vi "Language.vi"(6 "language cmd":T2, 8 "error in (no error)":errorcluster, 9 "Language":T3) -> (0 "error out":errorcluster, 3 "Language Data out":T1)   [LabVIEW 2015, in "AguaClara Library.lvlib"]
uses:
  AguaClara Library.lvlib
  Language.ctl
  language cmd.ctl
  Variable cluster.ctl
panel:
  in  "Language Data storage":T1=[{"Label.Text"="Quit", "Control Type"=0, "Numeric"=0.0, "Array"=[], "status"=FALSE, "Str Array"=[], "String"="", "unit"=""}, {"Label.Text"="Tab Control", "Control Type"=0, "Numeric"=0.0, "Array"=[], "status"=FALSE, "Str Array"=[], "String"="", "unit"=""}, {"Label.Text"="Help Button", "Control Type"=0, "Numeric"=0.0, "Array"=[], "status"=FALSE, "Str Array"=[], "String"="", "unit"=""}, {"Label.Text"="Logon", "Control Type"=0, "Numeric"=0.0, "Array"=[], "status"=FALSE, "Str Array"=[], "String"="", "unit"=""}, {"Label.Text"="Project List", "Control Type"=0, "Numeric"=0.0, "Array"=[], "status"=FALSE, "Str Array"=[], "String"="", "unit"=""}, {"Label.Text"="Project commands", "Control Type"=0, "Numeric"=0.0, "Array"=[], "status"=FALSE, "Str Array"=[], "String"="", "unit"=""}, {"Label.Text"="Log off", "Control Type"=0, "Numeric"=0.0, "Array"=[], "status"=FALSE, "Str Array"=[], "String"="", "unit"=""}, {"Label.Text"="Design Plant", "Control Type"=0, "Numeric"=0.0, "Array"=[], "status"=FALSE, "Str Array"=[], "String"="", "unit"=""}, {"Label.Text"="Project Info label", "Control Type"=0, "Numeric"=0.0, "Array"=[], "status"=FALSE, "Str Array"=[], "String"="", "unit"=""}, {"Label.Text"="Design Inputs Label", "Control Type"=0, "Numeric"=0.0, "Array"=[], "status"=FALSE, "Str Array"=[], "String"="", "unit"=""}, {"Label.Text"="MSG Design sent precity", "Control Type"=0, "Numeric"=0.0, "Array"=[], "status"=FALSE, "Str Array"=[], "String"="", "unit"=""}, {"Label.Text"="MSG Design sent postcity", "Control Type"=0, "Numeric"=0.0, "Array"=[], "status"=FALSE, "Str Array"=[], "String"="", "unit"=""}, {"Label.Text"="MSG Server unavailable", "Control Type"=0, "Numeric"=0.0, "Array"=[], "status"=FALSE, "Str Array"=[], "String"="", "unit"=""}, {"Label.Text"="Quit now", "Control Type"=0, "Numeric"=0.0, "Array"=[], "status"=FALSE, "Str Array"=[], "String"="", "unit"=""}, {"Label.Text"="Project Info", "Control Type"=0, "Numeric"=0.0, "Array"=[], "status"=FALSE, "Str Array"=[], "String"="", "unit"=""}, {"Label.Text"="Project Name", "Control Type"=0, "Numeric"=0.0, "Array"=[], "status"=FALSE, "Str Array"=[], "String"="", "unit"=""}, {"Label.Text"="City", "Control Type"=0, "Numeric"=0.0, "Array"=[], "status"=FALSE, "Str Array"=[], "String"="", "unit"=""}, {"Label.Text"="State", "Control Type"=0, "Numeric"=0.0, "Array"=[], "status"=FALSE, "Str Array"=[], "String"="", "unit"=""}, {"Label.Text"="Country", "Control Type"=0, "Numeric"=0.0, "Array"=[], "status"=FALSE, "Str Array"=[], "String"="", "unit"=""}, {"Label.Text"="Notes", "Control Type"=0, "Numeric"=0.0, "Array"=[], "status"=FALSE, "Str Array"=[], "String"="", "unit"=""}, {"Label.Text"="User Information", "Control Type"=0, "Numeric"=0.0, "Array"=[], "status"=FALSE, "Str Array"=[], "String"="", "unit"=""}, {"Label.Text"="First Name", "Control Type"=0, "Numeric"=0.0, "Array"=[], "status"=FALSE, "Str Array"=[], "String"="", "unit"=""}, {"Label.Text"="Last Name", "Control Type"=0, "Numeric"=0.0, "Array"=[], "status"=FALSE, "Str Array"=[], "String"="", "unit"=""}, {"Label.Text"="Email Address", "Control Type"=0, "Numeric"=0.0, "Array"=[], "status"=FALSE, "Str Array"=[], "String"="", "unit"=""}, {"Label.Text"="Organization", "Control Type"=0, "Numeric"=0.0, "Array"=[], "status"=FALSE, "Str Array"=[], "String"="", "unit"=""}, {"Label.Text"="Language", "Control Type"=0, "Numeric"=0.0, "Array"=[], "status"=FALSE, "Str Array"=[], "String"="", "unit"=""}, {"Label.Text"="AutoCAD File Type", "Control Type"=0, "Numeric"=0.0, "Array"=[], "status"=FALSE, "Str Array"=[], "String"="", "unit"=""}, {"Label.Text"="Project date", "Control Type"=0, "Numeric"=0.0, "Array"=[], "status"=FALSE, "Str Array"=[], "String"="", "unit"=""}, {"Label.Text"="Design Inputs", "Control Type"=0, "Numeric"=0.0, "Array"=[], "status"=FALSE, "Str Array"=[], "String"="", "unit"=""}, {"Label.Text"="Q.Plant", "Control Type"=0, "Numeric"=0.0, "Array"=[], "status"=FALSE, "Str Array"=[], "String"="", "unit"=""}, {"Label.Text"="C.CoagDoseMax", "Control Type"=0, "Numeric"=0.0, "Array"=[], "status"=FALSE, "Str Array"=[], "String"="", "unit"=""}, {"Label.Text"="C.CoagStock", "Control Type"=0, "Numeric"=0.0, "Array"=[], "status"=FALSE, "Str Array"=[], "String"="", "unit"=""}, {"Label.Text"="Ti.CoagStock", "Control Type"=0, "Numeric"=0.0, "Array"=[], "status"=FALSE, "Str Array"=[], "String"="", "unit"=""}, {"Label.Text"="EN.DrillSeries", "Control Type"=0, "Numeric"=0.0, "Array"=[], "status"=FALSE, "Str Array"=[], "String"="", "unit"=""}, {"Label.Text"="EN.TubeSeries", "Control Type"=0, "Numeric"=0.0, "Array"=[], "status"=FALSE, "Str Array"=[], "String"="", "unit"=""}, {"Label.Text"="EN.PipeSeries", "Control Type"=0, "Numeric"=0.0, "Array"=[], "status"=FALSE, "Str Array"=[], "String"="", "unit"=""}, {"Label.Text"="N.SedTanks", "Control Type"=0, "Numeric"=0.0, "Array"=[], "status"=FALSE, "Str Array"=[], "String"="", "unit"=""}, {"Label.Text"="N.SedBaysEst", "Control Type"=0, "Numeric"=0.0, "Array"=[], "status"=FALSE, "Str Array"=[], "String"="", "unit"=""}, {"Label.Text"="W.SedPlate", "Control Type"=0, "Numeric"=0.0, "Array"=[], "status"=FALSE, "Str Array"=[], "String"="", "unit"=""}, {"Label.Text"="L.SedPlateSheet", "Control Type"=0, "Numeric"=0.0, "Array"=[], "status"=FALSE, "Str Array"=[], "String"="", "unit"=""}, {"Label.Text"="T.SedPlate", "Control Type"=0, "Numeric"=0.0, "Array"=[], "status"=FALSE, "Str Array"=[], "String"="", "unit"=""}, {"Label.Text"="T.PlantWall", "Control Type"=0, "Numeric"=0.0, "Array"=[], "status"=FALSE, "Str Array"=[], "String"="", "unit"=""}, {"Label.Text"="H.FlocOption", "Control Type"=0, "Numeric"=0.0, "Array"=[], "status"=FALSE, "Str Array"=[], "String"="", "unit"=""}, {"Label.Text"="T.FlocBaffleRigidH", "Control Type"=0, "Numeric"=0.0, "Array"=[], "status"=FALSE, "Str Array"=[], "String"="", "unit"=""}, {"Label.Text"="T.ConcreteMin", "Control Type"=0, "Numeric"=0.0, "Array"=[], "status"=FALSE, "Str Array"=[], "String"="", "unit"=""}, {"Label.Text"="T.SedWeir", "Control Type"=0, "Numeric"=0.0, "Array"=[], "status"=FALSE, "Str Array"=[], "String"="", "unit"=""}, {"Label.Text"="T.FlocBaffleRigidV", "Control Type"=0, "Numeric"=0.0, "Array"=[], "status"=FALSE, "Str Array"=[], "String"="", "unit"=""}, {"Label.Text"="error out", "Control Type"=0, "Numeric"=0.0, "Array"=[], "status"=FALSE, "Str Array"=[], "String"="", "unit"=""}, {"Label.Text"="status", "Control Type"=0, "Numeric"=0.0, "Array"=[], "status"=FALSE, "Str Array"=[], "String"="", "unit"=""}, {"Label.Text"="code", "Control Type"=0, "Numeric"=0.0, "Array"=[], "status"=FALSE, "Str Array"=[], "String"="", "unit"=""}, {"Label.Text"="source", "Control Type"=0, "Numeric"=0.0, "Array"=[], "status"=FALSE, "Str Array"=[], "String"="", "unit"=""}, {"Label.Text"="File List", "Control Type"=0, "Numeric"=0.0, "Array"=[], "status"=FALSE, "Str Array"=[], "String"="", "unit"=""}, {"Label.Text"="Translate", "Control Type"=0, "Numeric"=0.0, "Array"=[], "status"=FALSE, "Str Array"=[], "String"="", "unit"=""}, {"Label.Text"="CheckOut ADT", "Control Type"=0, "Numeric"=0.0, "Array"=[], "status"=FALSE, "Str Array"=[], "String"="", "unit"=""}, {"Label.Text"="ADT version", "Control Type"=0, "Numeric"=0.0, "Array"=[], "status"=FALSE, "Str Array"=[], "String"="", "unit"=""}, {"Label.Text"="Choose Server", "Control Type"=0, "Numeric"=0.0, "Array"=[], "status"=FALSE, "Str Array"=[], "String"="", "unit"=""}, {"Label.Text"="design server", "Control Type"=0, "Numeric"=0.0, "Array"=[], "status"=FALSE, "Str Array"=[], "String"="", "unit"=""}, {"Label.Text"="Restart ADT", "Control Type"=0, "Numeric"=0.0, "Array"=[], "status"=FALSE, "Str Array"=[], "String"="", "unit"=""}, {"Label.Text"="Create New Project", "Control Type"=0, "Numeric"=0.0, "Array"=[], "status"=FALSE, "Str Array"=[], "String"="", "unit"=""}, {"Label.Text"="Edit Project", "Control Type"=0, "Numeric"=0.0, "Array"=[], "status"=FALSE, "Str Array"=[], "String"="", "unit"=""}, {"Label.Text"="Delete Project", "Control Type"=0, "Numeric"=0.0, "Array"=[], "status"=FALSE, "Str Array"=[], "String"="", "unit"=""}, {"Label.Text"="Valid User Options", "Control Type"=0, "Numeric"=0.0, "Array"=[], "status"=FALSE, "Str Array"=[], "String"="", "unit"=""}, {"Label.Text"="Okay Button", "Control Type"=0, "Numeric"=0.0, "Array"=[], "status"=FALSE, "Str Array"=[], "String"="", "unit"=""}, {"Label.Text"="logon status", "Control Type"=0, "Numeric"=0.0, "Array"=[], "status"=FALSE, "Str Array"=[], "String"="", "unit"=""}, {"Label.Text"="valid user", "Control Type"=0, "Numeric"=0.0, "Array"=[], "status"=FALSE, "Str Array"=[], "String"="", "unit"=""}, {"Label.Text"="User Information out", "Control Type"=0, "Numeric"=0.0, "Array"=[], "status"=FALSE, "Str Array"=[], "String"="", "unit"=""}, {"Label.Text"="Cancel Button", "Control Type"=0, "Numeric"=0.0, "Array"=[], "status"=FALSE, "Str Array"=[], "String"="", "unit"=""}, {"Label.Text"="User Index out", "Control Type"=0, "Numeric"=0.0, "Array"=[], "status"=FALSE, "Str Array"=[], "String"="", "unit"=""}, {"Label.Text"="User Index in", "Control Type"=0, "Numeric"=0.0, "Array"=[], "status"=FALSE, "Str Array"=[], "String"="", "unit"=""}, {"Label.Text"="New Account", "Control Type"=0, "Numeric"=0.0, "Array"=[], "status"=FALSE, "Str Array"=[], "String"="", "unit"=""}, {"Label.Text"="Update User Info", "Control Type"=0, "Numeric"=0.0, "Array"=[], "status"=FALSE, "Str Array"=[], "String"="", "unit"=""}, {"Label.Text"="Language Data", "Control Type"=0, "Numeric"=0.0, "Array"=[], "status"=FALSE, "Str Array"=[], "String"="", "unit"=""}, {"Label.Text"="OK Button", "Control Type"=0, "Numeric"=0.0, "Array"=[], "status"=FALSE, "Str Array"=[], "String"="", "unit"=""}, {"Label.Text"="Language Data out", "Control Type"=0, "Numeric"=0.0, "Array"=[], "status"=FALSE, "Str Array"=[], "String"="", "unit"=""}, {"Label.Text"="updated", "Control Type"=0, "Numeric"=0.0, "Array"=[], "status"=FALSE, "Str Array"=[], "String"="", "unit"=""}, {"Label.Text"="Table Control", "Control Type"=0, "Numeric"=0.0, "Array"=[], "status"=FALSE, "Str Array"=[], "String"="", "unit"=""}, {"Label.Text"="Load from VNG", "Control Type"=0, "Numeric"=0.0, "Array"=[], "status"=FALSE, "Str Array"=[], "String"="", "unit"=""}, {"Label.Text"="Design Inputs out", "Control Type"=0, "Numeric"=0.0, "Array"=[], "status"=FALSE, "Str Array"=[], "String"="", "unit"=""}, {"Label.Text"="Project Info out", "Control Type"=0, "Numeric"=0.0, "Array"=[], "status"=FALSE, "Str Array"=[], "String"="", "unit"=""}, {"Label.Text"="canceled", "Control Type"=0, "Numeric"=0.0, "Array"=[], "status"=FALSE, "Str Array"=[], "String"="", "unit"=""}, {"Label.Text"="Reset to Default", "Control Type"=0, "Numeric"=0.0, "Array"=[], "status"=FALSE, "Str Array"=[], "String"="", "unit"=""}, {"Label.Text"="Basic Inputs", "Control Type"=0, "Numeric"=0.0, "Array"=[], "status"=FALSE, "Str Array"=[], "String"="", "unit"=""}, {"Label.Text"="Floc tank depth controls", "Control Type"=0, "Numeric"=0.0, "Array"=[], "status"=FALSE, "Str Array"=[], "String"="", "unit"=""}, {"Label.Text"="HW.FlocEnd", "Control Type"=0, "Numeric"=0.0, "Array"=[], "status"=FALSE, "Str Array"=[], "String"="", "unit"=""}, {"Label.Text"="HW.FlocEndDepth", "Control Type"=0, "Numeric"=0.0, "Array"=[], "status"=FALSE, "Str Array"=[], "String"="", "unit"=""}, {"Label.Text"="Language data", "Control Type"=0, "Numeric"=0.0, "Array"=[], "status"=FALSE, "Str Array"=[], "String"="", "unit"=""}, {"Label.Text"="error in", "Control Type"=0, "Numeric"=0.0, "Array"=[], "status"=FALSE, "Str Array"=[], "String"="", "unit"=""}, {"Label.Text"="VI controls", "Control Type"=0, "Numeric"=0.0, "Array"=[], "status"=FALSE, "Str Array"=[], "String"="", "unit"=""}, {"Label.Text"="Progress bar", "Control Type"=0, "Numeric"=0.0, "Array"=[], "status"=FALSE, "Str Array"=[], "String"="", "unit"=""}]
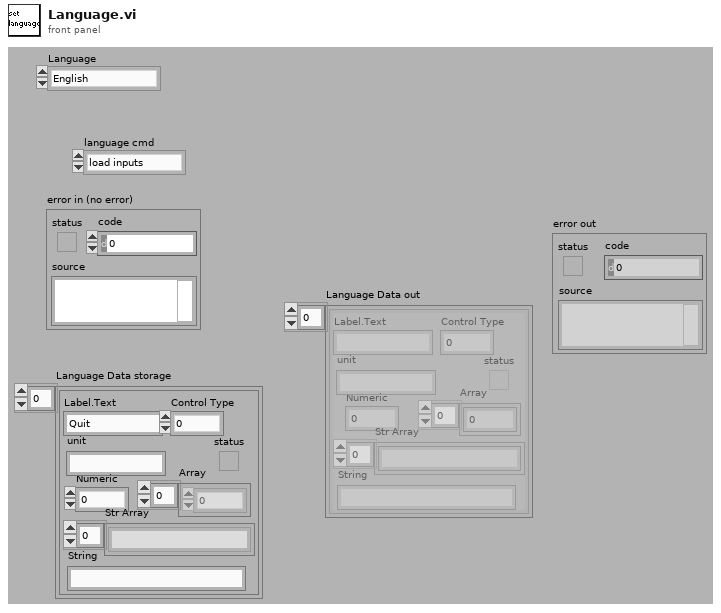
[diagram p1: front panel]
types:
  T1 = typedef "Variable cluster.ctl" = cluster{"Label.Text":string, "Control Type":u32, "Numeric":dbl, "Array":dbl[], "status":bool, "Str Array":string[], "String":string, "unit":string}[]
  T2 = typedef "AguaClara Library.lvlib/language cmd.ctl" = enum16{"load inputs", "choose language", "translate", "load storage variable from file"}
  T3 = typedef "AguaClara Library.lvlib/Language.ctl" = enum16{"English", "Español", "French"}
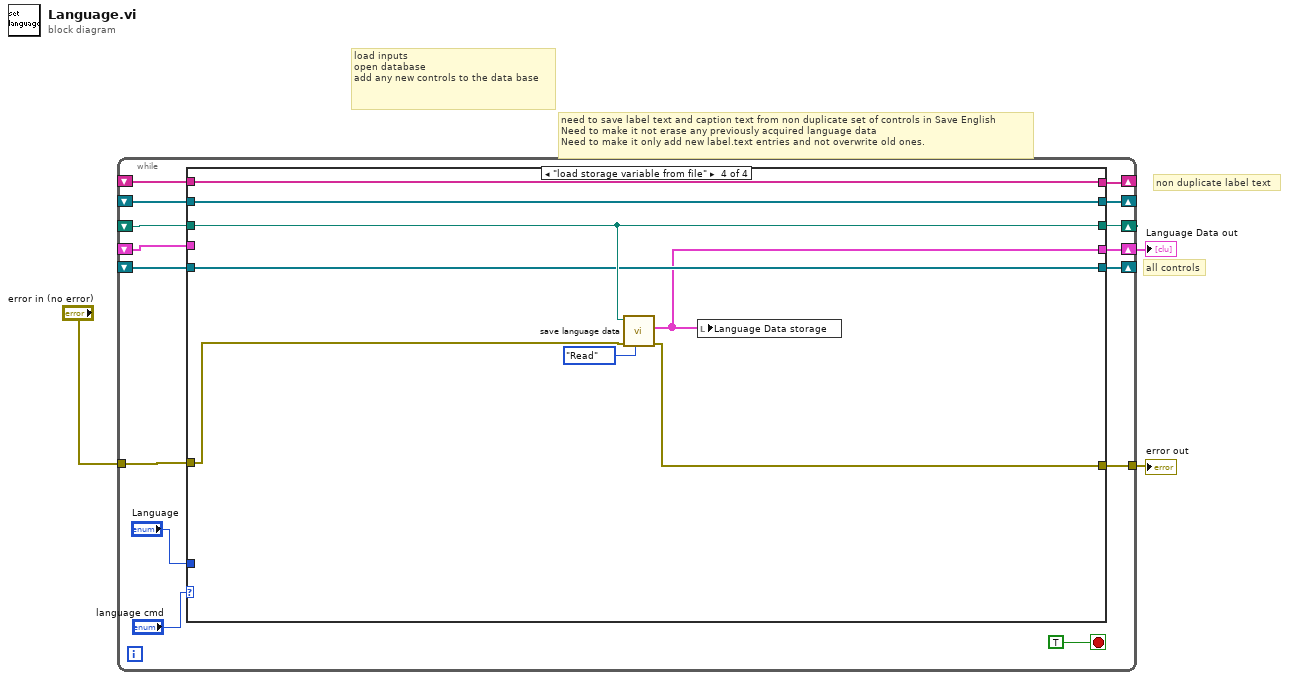
[diagram p0: block diagram]
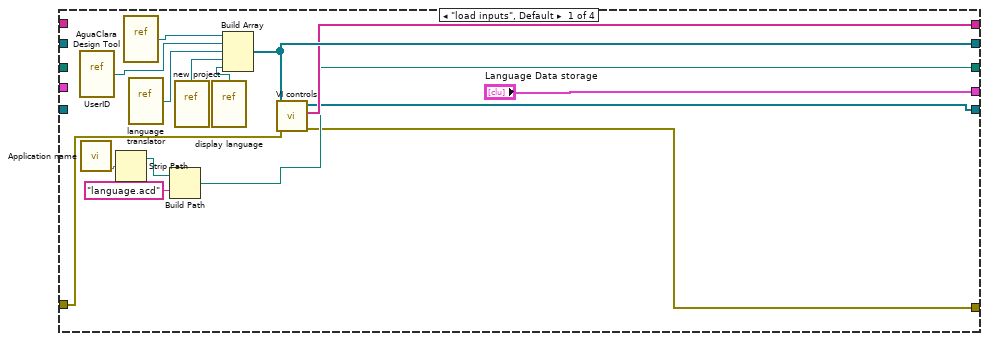
[diagram p2: hidden frame]
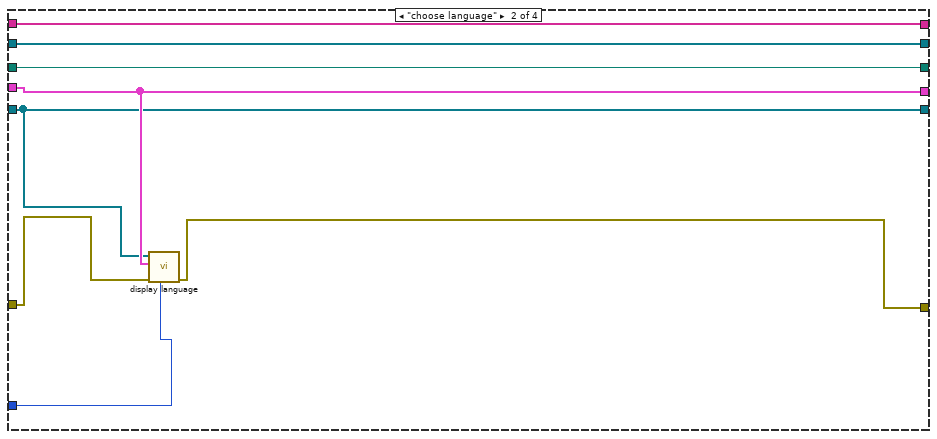
[diagram p3: hidden frame]
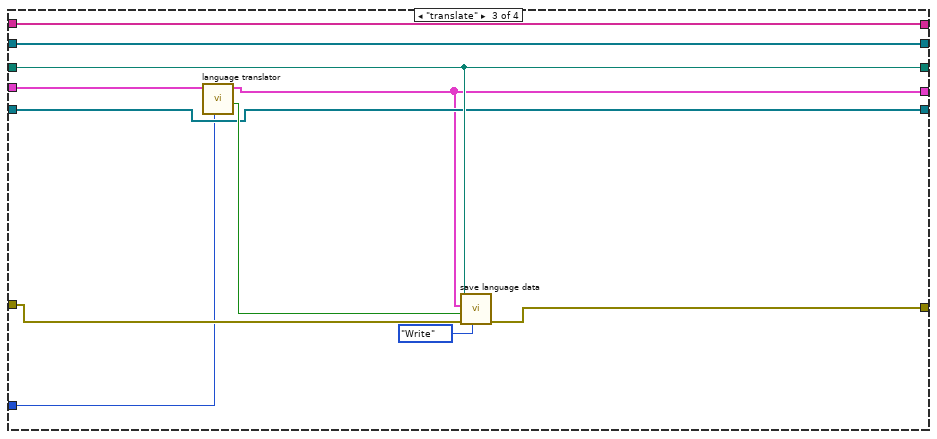
[diagram p4: hidden frame]
diagram:
  # "non duplicate label text"
  # "load inputs\nopen database\nadd any new controls to the data base"
  # "need to save label text and caption text from non duplicate set of controls in Save English \nNeed to make it not erase any previously acquired language data\nNeed to make it only add new label.text entries and not overwrite old ones."
  # "all controls"
  n1 = while {
    tunnel: "error in (no error)" -> [w16]
    tunnel: [w18] -> w2
    shift-right: [w17] -> _
    shift-left: _ -> [w13]
    shift-right: [w12] -> _
    shift-left: _ -> [w11]
    shift-right: [w10] -> w1
    shift-left: _ -> [w9]
    shift-right: [w8] -> _
    shift-left: _ -> [w7]
    shift-right: [w5] -> _
    shift-left: _ -> [w4]
    stop <- TRUE stop-if-true
    n2 = case shown="\"load storage variable from file\"" "language cmd" {
      tunnel: [w19 w34 w46 w55] -> w18
      tunnel: [w29 w40 w52 w59] -> w17
      tunnel: w16 -> [w28 w35 w49 w56]
      tunnel: w13 -> [_ w40 w52 w59]
      tunnel: [w25 w41 w48 w58] -> w12
      tunnel: w11 -> [_ w41 w48 w58]
      tunnel: ["Language Data storage" w38 w45 w53] -> w10
      tunnel: w9 -> [_ w38 w51 _]
      tunnel: [w26 w37 w47 w54] -> w8
      tunnel: w7 -> [_ w37 w47 w54]
      tunnel: "Language" -> [_ w36 w43 _]
      tunnel: [w27 w39 w44 w60] -> w5
      tunnel: w4 -> [_ w39 w44 w60]
      frame "load inputs", Default {
        n3 = vi-ref "UserID.vi"() -> (w31:refnum<vi>)
        n4 = call "Application name.vi"() -> (0:w24)  [unwired: 4 in, 3 out]
        n5 = Strip Path(path=w24) -> (stripped path=w23:path)  [unwired: 1 out]
        n6 = vi-ref "AguaClara Design Tool.vi"() -> (w30:refnum<vi>)
        n7 = vi-ref "language translator.vi"() -> (w32:refnum<vi>)
        n8 = Build Path(base path=w23, name or relative path="language.acd") -> (appended path=w25:path)
        n9 = vi-ref "new project.vi"() -> (w22:refnum<vi>)
        n10 = vi-ref "display language.vi"() -> (w21:refnum<vi>)
        n11 = Build Array(w30, w31, w32, w22, w21) -> (w29:refnum<vi>[])
        n12 = call "VI controls.vi"("error in (no error)"=w28, "VI refnums"=w29) -> ("error out"=w19:errorcluster, "all Label text"=w27:string[], "VI controls"=w26:refnum<vi>[])  [unwired: 7 in]
      }
      frame "choose language" {
        n13 = call "display language.vi"("Language"=w36, "error in"=w35, "Language data"=w38, "VI controls"=w37) -> ("error out"=w34:errorcluster)  [unwired: 7 in]
      }
      frame "translate" {
        n14 = call "language translator.vi"("Language"=w43, "Language Data"=w51) -> ("updated"=w50:bool, "Language Data out"=w45:T1)  [unwired: 8 in]
        n15 = call "save language data.vi"("R/W"=enum16{"Read", "Write"}."Write", "error in (no error)"=w49, "updated"=w50, "Language Data"=w45, "appended path"=w48) -> ("error out"=w46:errorcluster)  [unwired: 5 in, 1 out]
      }
      frame "load storage variable from file" {
        n16 = call "save language data.vi"("R/W"=enum16{"Read", "Write"}."Read", "error in (no error)"=w56, "appended path"=w58) -> ("error out"=w55:errorcluster, "Language Data out"=w53:T1)  [unwired: 7 in]
        n17 = local write "Language Data storage"(w53) -> ()
      }
    }
  }
  "error out" <- w2
  "Language Data out" <- w1
